vi "u-blox 5 Series Acquire and Chart GPS Data.vi"() -> ()   [LabVIEW 2009]
doc: "This example shows how to acquire GPS data from a u-blox 5 GPS device with KickStart."
panel:
  out "Altitude Chart":waveform(dbl)(graph)
  out "Speed Chart":waveform(dbl)(graph)
  in  "?":bool
  out "Position":cluster{dbl, dbl}[](graph)
  out "Time":timestamp
  in  "Reset Before Reading (False)":bool
  in  "VISA resource name":refnum<visa-resource-name>
  # "(c) 2009 National Instruments.  ALL RIGHTS RESERVED."
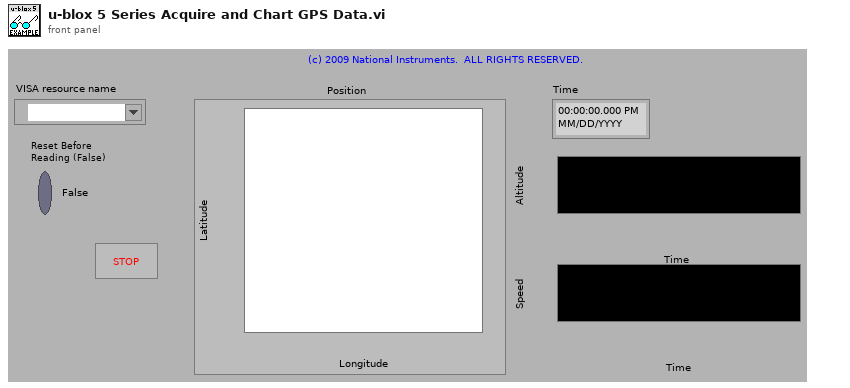
[diagram p1: front panel]
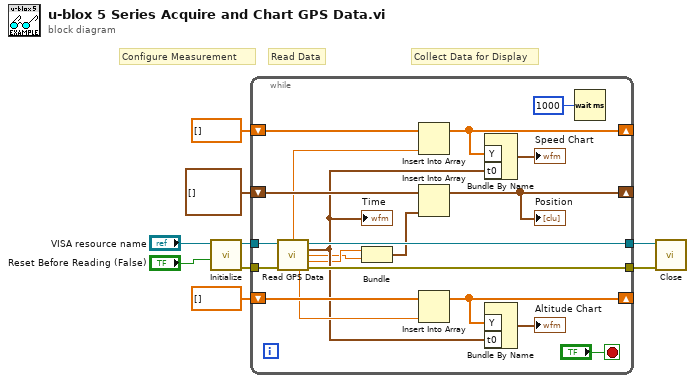
[diagram p0: block diagram]
diagram:
  # "Collect Data for Display"
  # "Read Data"
  # "Configure Measurement"
  n1 = call "Initialize.vi"("Reset (False)"="Reset Before Reading (False)", "VISA resource name"="VISA resource name") -> ("error out"=w7:errorcluster, "VISA resource name out"=w6:refnum<visa-resource-name>)  [unwired: 8 in]
  n2 = while {
    tunnel: w7 -> [w29]
    tunnel: w6 -> [w28]
    tunnel: [w27] -> w5
    tunnel: [w26] -> w4
    shift-right: [w21] -> _
    shift-left: cluster{dbl, dbl}[] [] ("Position") -> [w22]
    shift-right: [w18] -> _
    shift-left: dbl[] [] -> [w19]
    shift-right: [w14] -> _
    shift-left: dbl[] [] -> [w16]
    stop <- "?" stop-if-true
    n3 = call "Read GPS Data.vi"("VISA resource name"=w28, "error in (no error)"=w29) -> ("Speed Over Ground (knots)"=w20:dbl, "VISA resource name out"=w27:refnum<visa-resource-name>, "Time Stamp"=w12:timestamp, "Latitude (°)"=w10:dbl, "Longitude (°)"=w11:dbl, "Altitude (m)"=w15:dbl, "error out"=w26:errorcluster)  [unwired: 6 in, 1 out]
    "Time" <- w12
    n4 = Bundle("Longitude (°)"=w11, "Latitude (°)"=w10) -> (w23:cluster{"Longitude (°)":dbl, "Latitude (°)":dbl})  [unwired: 1 in]
    n5 = Insert Into Array(array=w19, new element=w20) -> (w18:dbl[])  [unwired: 1 in]
    n6 = Insert Into Array(array=w22, new element=w23) -> (w21:cluster{dbl, dbl}[])  [unwired: 1 in]
    "Position" <- w21
    n7 = Insert Into Array(array=w16, new element=w15) -> (w14:dbl[])  [unwired: 1 in]
    n8 = Bundle By Name("Y"=w18, "t0"=w12) -> (→"Speed Chart":waveform(dbl))  [unwired: 1 in]
    n9 = Bundle By Name("Y"=w14, "t0"=w12) -> (→"Altitude Chart":waveform(dbl))  [unwired: 1 in]
    n10 = Wait (ms)(milliseconds to wait=u32 1000) -> ()  [unwired: 1 out]
  }
  n11 = call "Close.vi"("error in (no error)"=w4, "VISA resource name"=w5) -> ()  [unwired: 9 in, 1 out]
